vi "RTG Example_reduced_20230830.vi"() -> ()   [LabVIEW 2020]
doc: "This example illustrates how to use the RTG local API to control the RTG."
uses:
  <vilib>/RTG/API/ip/common/host-types/Target Configuration.ctl
  <vilib>/RTG/API/ip/common/host-types/Synchronization - Host.ctl
  <vilib>/RTG/API/ip/common/host-types/Synchronization Mode - Host.ctl
  <vilib>/RTG/API/ip/common/host-types/Basic Target - Host.ctl
  <vilib>/RTG/API/interface/public/State.ctl
  <vilib>/RTG/coprocessor/host/RTG Coprocessor Link Interface/Public/Coprocessor Status.ctl
  <vilib>/RTG/API/ip/common/host-types/Target Motion Parameters.ctl
  <vilib>/RTG/API/ip/common/host-types/Single Target Motion Parameters.ctl
  <vilib>/RTG/API/interface/public/Coprocessor Link Status.ctl
  support/Options - API Mode.ctl
  support/Options - Calibration.ctl
  support/Options - Remote.ctl
  <vilib>/Utility/error.llb/Error Cluster From Error Code.vi
  <vilib>/rvi/errors/niLvFpgaAdjustHostInterfaceError.vi
  <vilib>/rvi/interface/nirviReadWriteControl/nirviReadWriteControl.xnode
  <vilib>/RTG/API/interface/NI-RTG Interface.lvclass
  <vilib>/RTG/coprocessor/host/RTG Coprocessor Link Interface/RTG Coprocessor Link Interface.lvclass
  <vilib>/RTG/API/ip/common/host-types/Host Data Types v1.lvlib
  RTG Examples.lvlib
  NiFpgaLv.dll
  <vilib>/rvi/interface/Simulation/niFpgaSimulationCallBeginRW.vi
panel:
  out "RTG Status":string
  out "RTG State":T1
  in  "tab":T2(tab)
  in  "abort system self cal":bool
  in  "Set PRIs":bool
  in  "PRI (s)":dbl[](array[numeric]) format="%#_6p"
  in  "Calibrate":bool=TRUE
  in  "Instrument Names":string[](array[string])=["5831_0"]
  in  "Center Freqeuncies (Hz)":dbl[](array[numeric])=[5500000000.0] format="%#_6p"
  in  "Reference Levels (dBm)":dbl[](array[numeric])=[0.0]
  in  "mmWave Radio Heads Enable":bool[](array[boolean])
  in  "External Delay (s)":dbl[](array[numeric]) format="%#_6p"
  in  "External Attenuations (dB)":dbl[](array[numeric])
  in  "Offset Frequencies (Hz)":dbl[](array[numeric]) format="%#_6p"
  out "Error Out":errorcluster caption="error out"
  in  "Coprocessor Names":string[](array[string])
  out "Versions":string[](array[string])
  out "Max Common Attenuations (dB)":dbl[](array[numeric])
  out "Min Common Attenuations (dB)":dbl[](array[numeric])
  out "Min Latencies (s)":dbl[](array[numeric]) format="%#_6p"
  in  "configure common attenuation":bool
  in  "Common Attenuation (dB)":dbl
  in  "set hardware trigger":bool
  in  "send target motion":bool
  in  "Auto Send Software Trigger":bool
  in  "Prepend Software Trigger":bool
  in  "send files":bool
  in  "Target Configuration Files":path[](array[path])
  in  "pulse detection calibration":bool
  in  "send target config":bool
  in  "send sw trigger":bool
  in  "start rtg":bool
  in  "stop rtg":bool
  in  "abort":bool
  in  "Target Configuration":T3 {"rtg targets"."time offset (s)" format="%#_6p"; "rtg targets"."doppler" format="%#_6p"}
  in  "Device Index":i32
  in  "Target Motion Parameters":T7={"target motions"=[{"target enable"=FALSE, "start time offset (s)"=-1e-09, "time offset rate of change (s/s)"=0.001, "start attenuation (dB)"=0.0, "attenuation rate of change (dB/s)"=0.0, "start frequency shift (Hz)"=0.0, "frequency shift rate of change (Hz/sec)"=0.0}], "scenario duration (s)"=67.0, "configuration update rate(Hz)"=15000.0} {"configuration update rate(Hz)" format="%#_6p"; "target motions"."frequency shift rate of change (Hz/sec)" format="%#_6p"; "target motions"."start frequency shift (Hz)" format="%#_6p"; "target motions"."time offset rate of change (s/s)" format="%#_6p"; "target motions"."start time offset (s)" format="%#_6p"}
  in  "Data Path Enable":bool=TRUE
  in  "Hardware Trigger":string="PXI_Trig7"
  out "Device Index vs Trigger Count":i32[][](array[numeric])
  out "coprocessor link status":T9[](array[typedef])
  out "rtg link status":T10[](array[typedef])
  # "Coprocessor"
  # "Configuration Files and Target Motion"
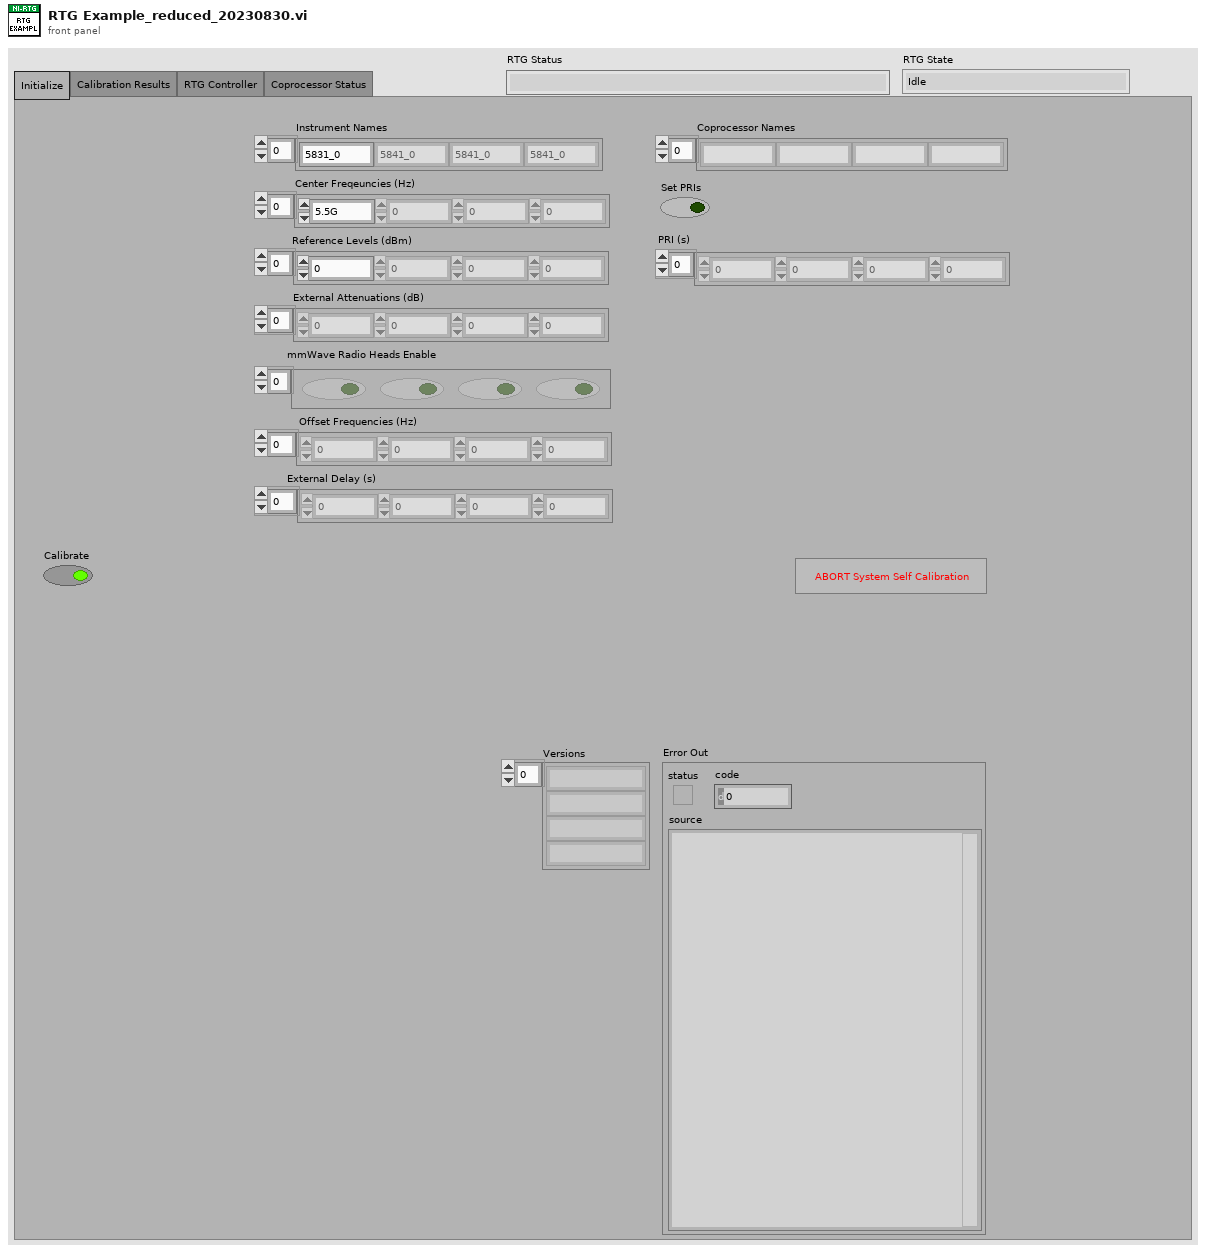
[diagram p1: front panel]
types:
  T1 = typedef "NI-RTG v1.lvlib/NI-RTG Interface.lvclass/State.ctl" = enum16{"Idle", "Inactive", "Active", "System Self Calibration"}
  T2 = enum32{"Initialize", "Calibration Results", "RTG Controller", "Coprocessor Status"}
  T3 = typedef "Host Data Types v1.lvlib/Target Configuration.ctl" = cluster{"synchronization":T4, "rtg targets":T6[]}
  T4 = typedef "Host Data Types v1.lvlib/Synchronization - Host.ctl" = cluster{"synch mode":T5, "time offset (s)":dbl}
  T5 = typedef "Host Data Types v1.lvlib/Synchronization Mode - Host.ctl" = enum16{"Software Trigger", "Hardware Trigger", "Time Offset Relative to First", "Time Offset Relative to Last", "Pulse Rising Edge", "Pulse Falling Edge"}
  T6 = typedef "Host Data Types v1.lvlib/Basic Target - Host.ctl" = cluster{"time offset (s)":dbl, "attenuaton (dB)":dbl, "doppler":dbl, "target enable":bool, "relative velocity enable":bool}
  T7 = typedef "Host Data Types v1.lvlib/Target Motion Parameters.ctl" = cluster{"target motions":T8[], "scenario duration (s)":dbl, "configuration update rate(Hz)":dbl}
  T8 = typedef "Host Data Types v1.lvlib/Single Target Motion Parameters.ctl" = cluster{"target enable":bool, "start time offset (s)":dbl, "time offset rate of change (s/s)":dbl, "start attenuation (dB)":dbl, "attenuation rate of change (dB/s)":dbl, "start frequency shift (Hz)":dbl, "frequency shift rate of change (Hz/sec)":dbl}
  T9 = typedef "RTG Coprocessor Link Interface v1 Host.lvlib/RTG Coprocessor Link Interface.lvclass/Coprocessor Status.ctl" = cluster{"tx read count":u64, "tx read overflow":bool, "rx read count":u64, "rx read overflow":bool}
  T10 = typedef "NI-RTG v1.lvlib/NI-RTG Interface.lvclass/Coprocessor Link Status.ctl" = cluster{"task name":string, "device name":string, "hard error":bool, "soft error":bool, "channel up":bool, "system reset":bool}
  T11 = typedef "RTG Examples.lvlib/Options - API Mode.ctl" = enum16{"Local", "Remote"}
  T12 = typedef "RTG Examples.lvlib/Options - Calibration.ctl" = cluster{"enable internal loopback  ":bool, "enable overwrite cal data  ":bool, "enable save cal data           ":bool, "disable self cal range          ":bool}
  T13 = typedef "RTG Examples.lvlib/Options - Remote.ctl" = cluster{"ip address":string, "port":string, "certificate path":path, "timeout (ms)":i32}
  T14 = cluster{"API Mode":T11, "Calibration Options":T12, "Remote Options":T13, "ini file path":path}
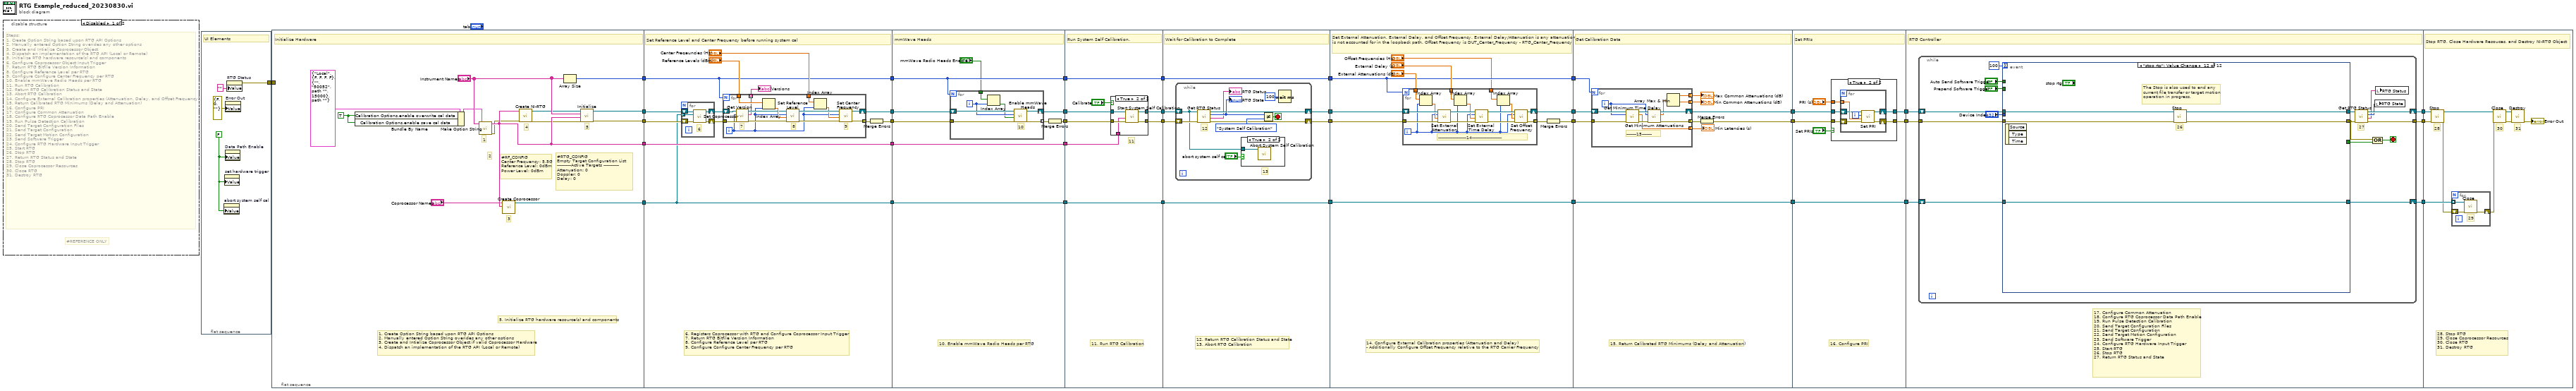
[diagram p0: block diagram]
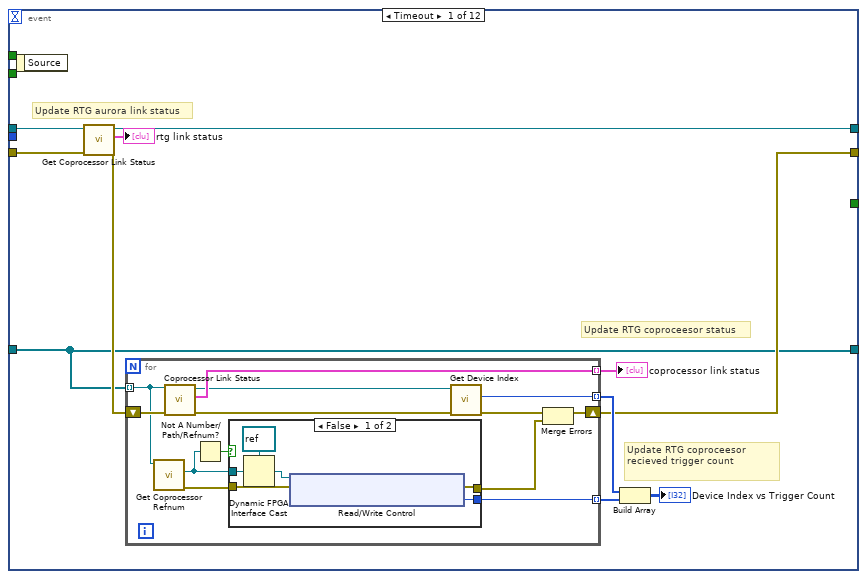
[diagram p6: hidden frame]
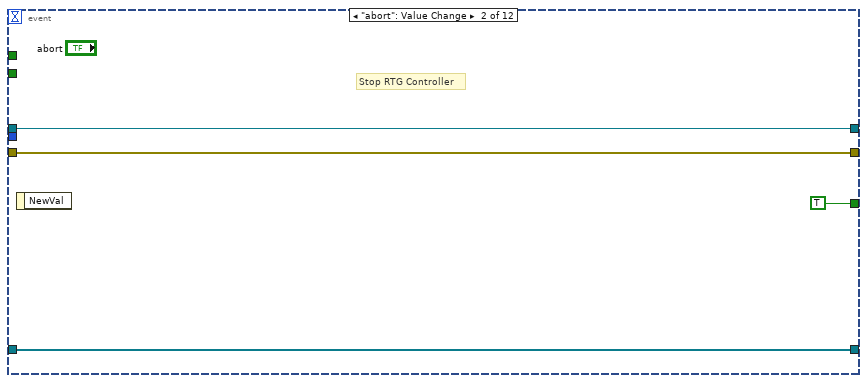
[diagram p8: hidden frame]
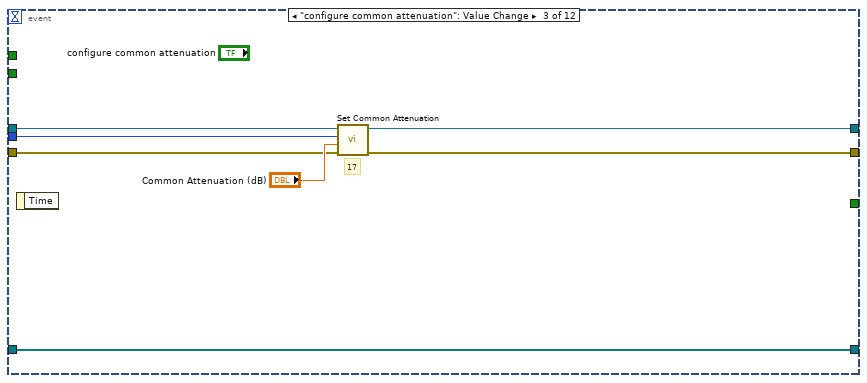
[diagram p9: hidden frame]
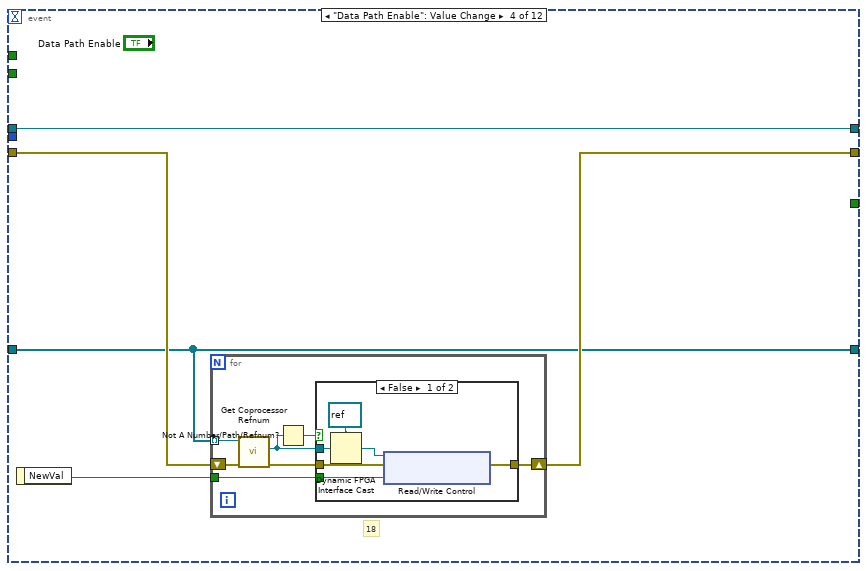
[diagram p10: hidden frame]
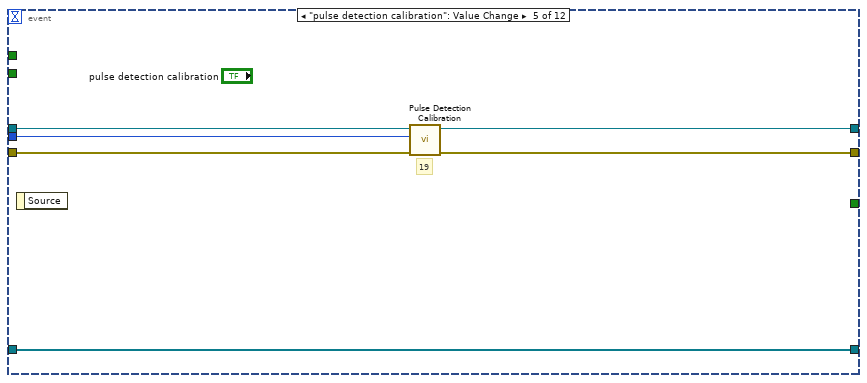
[diagram p12: hidden frame]
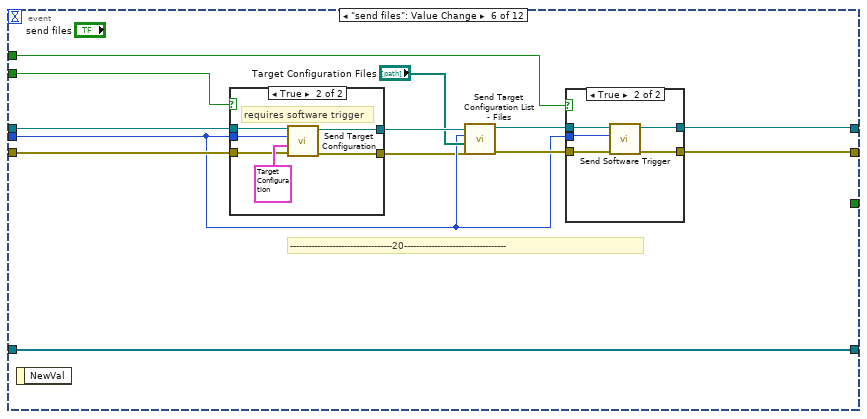
[diagram p13: hidden frame]
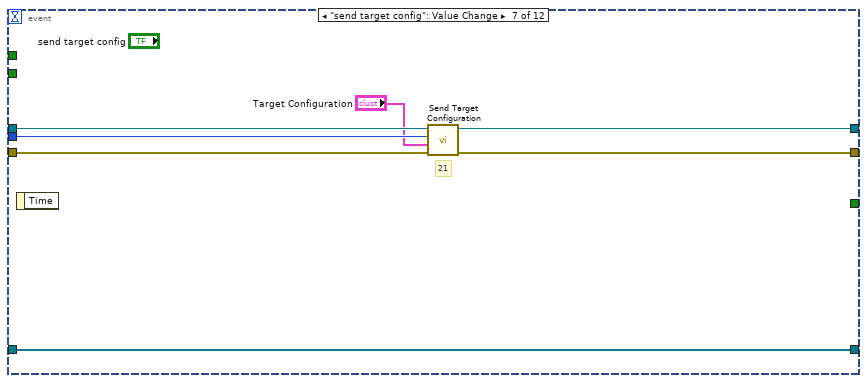
[diagram p16: hidden frame]
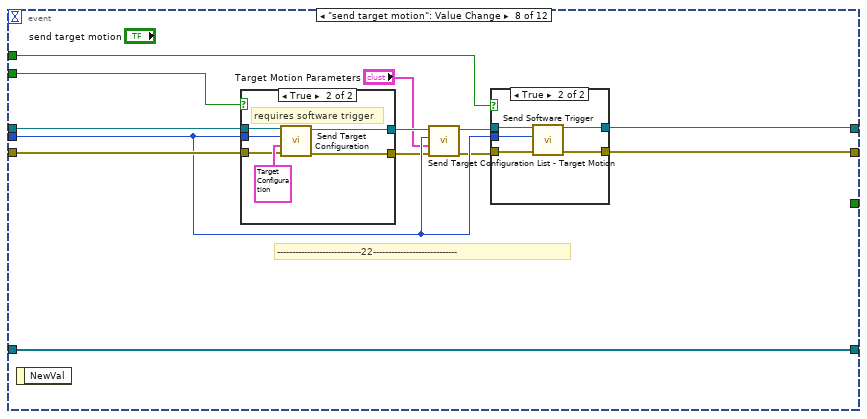
[diagram p17: hidden frame]
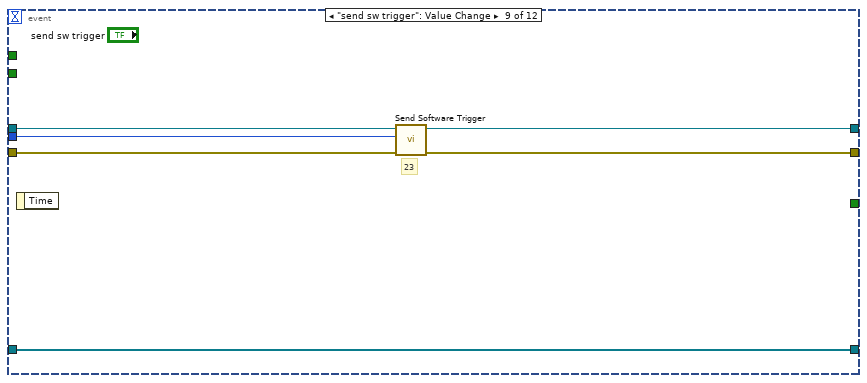
[diagram p20: hidden frame]
diagram:
  n1 = disable-structure shown="Disabled" {
    frame Disabled {
      # "#REFERENCE ONLY"
      # "Steps:\n1. Create Option String based upon RTG API Options\n2. Manually entered Option String overides any other options\n3. Create and Intialize Coprocessor Object\n4. Dispatch an implementation of the RTG API (Local or Remote)\n5. Initialize RTG hardware resource(s) and components\n6. Configure Coprocessor Object Input Trigger\n7. Return RTG Bitfile Version Information\n8. Configure Reference Level per RTG\n9. Configure Configure Center Frequency per RTG\n10. Enable mmWave Radio Heads per RTG\n11. Run RTG Calibration\n12. Return RTG Calibration Status and State\n13. Abort RTG Calibration\n14. Configure External Calibration properties (Attenuation, Delay, and Offset Frequency)\n15. Return Calibrated RTG Minimums (Delay and Attenuation)\n16. Configure PRI\n17. Configure Common Attenuation\n18. Configure RTG Coprocessor Data Path Enable \n19. Run Pulse Detection Calibration\n20. Send Target Configuration Files\n21. Send Target Configuration\n22. Send Target Motion Configuration\n23. Send Software Trigger\n24. Configure RTG Hardware Input Trigger\n25. Start RTG\n26. Stop RTG\n27. Return RTG Status and State\n28. Stop RTG\n29. Close Coprocessor Resources\n30. Close RTG\n31. Destroy RTG"
    }
    frame Enabled {
    }
  }
  n2 = flat-sequence {
    tunnel: [w40] -> w7
    frame #0 {
      w38 = FALSE ("bitfiles loaded")
      # "UI Elements"
      n3 = property on="abort system self cal" class="Bool (strict)"("Value"=w38) -> ()  [unwired: 2 in, 2 out]
      n4 = property on="set hardware trigger" class="Bool (strict)"("Value"=w38) -> ()  [unwired: 2 in, 2 out]
      n5 = property on="Data Path Enable" class="Bool (strict)"("Value"=w38) -> ()  [unwired: 2 in, 2 out]
      n6 = property on="Error Out" class="Clust (strict)"("Value"=errorcluster {"status"=FALSE, "code"=0, "source"=""} ("error out")) -> ()  [unwired: 2 in, 2 out]
      n7 = property on="RTG Status" class="Str"("Value"="" ("rtg status")) -> (error out=w40:errorcluster)  [unwired: 2 in, 1 out]
    }
  }
  n8 = flat-sequence {
    tunnel: [w49] -> w37
    tunnel: [w47] -> w36
    tunnel: [w54] -> w35
    tunnel: [w52] -> w17
    tunnel: [w51] -> w14
    tunnel: w7 -> [_]
    tunnel: w37 -> [w58]
    tunnel: w36 -> [w55]
    tunnel: [w65] -> w29
    tunnel: [w63] -> w27
    tunnel: w35 -> [w62]
    tunnel: [w62] -> w25
    tunnel: w17 -> [w61]
    tunnel: [w61] -> w16
    tunnel: w14 -> [w57]
    tunnel: [w57] -> w12
    tunnel: w29 -> [w94]
    tunnel: [w89] -> w28
    tunnel: w27 -> [w93]
    tunnel: [w91] -> w26
    tunnel: w25 -> [w95]
    tunnel: [w95] -> w24
    tunnel: w16 -> [w88]
    tunnel: [w88] -> w15
    tunnel: [w87] -> w13
    tunnel: w12 -> [w87]
    tunnel: w28 -> [w110]
    tunnel: w26 -> [w109]
    tunnel: [w107] -> w23
    tunnel: [w108] -> w22
    tunnel: w24 -> [w108]
    tunnel: [w106] -> w20
    tunnel: w15 -> [w105]
    tunnel: w13 -> [w103]
    tunnel: [w103] -> w11
    tunnel: w23 -> [w122]
    tunnel: w22 -> [w123]
    tunnel: [w123] -> w21
    tunnel: w20 -> [w121]
    tunnel: [w120] -> w19
    tunnel: [w119] -> w18
    tunnel: w11 -> [w118]
    tunnel: [w118] -> w10
    tunnel: [w141] -> w32
    tunnel: [w140] -> w31
    tunnel: [w139] -> w30
    tunnel: w21 -> [w139]
    tunnel: w19 -> [w138]
    tunnel: w18 -> [w137]
    tunnel: w10 -> [w135]
    tunnel: [w135] -> w9
    tunnel: w32 -> [w167]
    tunnel: [w166] -> w6
    tunnel: w31 -> [w169]
    tunnel: [w165] -> w4
    tunnel: w30 -> [w161]
    tunnel: w9 -> [w160]
    tunnel: [w160] -> w2
    tunnel: w6 -> [w185]
    tunnel: [w184] -> w5
    tunnel: w4 -> [w183]
    tunnel: [w182] -> w3
    tunnel: w2 -> [w187]
    tunnel: [w187] -> w1
    tunnel: w5 -> [w206]
    tunnel: w3 -> [w205]
    tunnel: [w204] -> w34
    tunnel: [w203] -> w33
    tunnel: w1 -> [w202]
    tunnel: [w201] -> w8
    tunnel: w34 -> [w395]
    tunnel: w33 -> [w389]
    tunnel: w8 -> [w390]
    frame #0 {
      w42 = TRUE ("Calibration Options.enable overwrite cal data")
      # "1. Create Option String based upon RTG API Options\n2. Manually entered Option String overides any other options\n3. Create and Intialize Coprocessor Object if valid Coprocessor Hardware\n4. Dispatch an implementation of the RTG API (Local or Remote)"
      # "4"
      # "3"
      # "2"
      # "1"
      # "5. Initialize RTG hardware resource(s) and components"
      # "5"
      # "#RTG_CONFIG\nEmpty Target Configuration List\n----------Active Targets -----------\nAttenuation: 0\nDoppler: 0\nDelay: 0"
      # "#RF_CONFIG\nCenter Frequency: 5.5G\nReference Level: 0dBm\nPower Level: 0dBm"
      # "Initialize Hardware"
      n9 = Bundle By Name(cluster=T14 {"API Mode"=enum."Local", "Calibration Options"={"enable internal loopback  "=FALSE, "enable overwrite cal data  "=FALSE, "enable save cal data           "=FALSE, "disable self cal range          "=FALSE}, "Remote Options"={"ip address"="", "port"="50052", "certificate path"=path "", "timeout (ms)"=15000}, "ini file path"=path ""} ("RTG API Options"), "Calibration Options.enable overwrite cal data"=w42, "Calibration Options.enable save cal data"=w42) -> (w43:T14)
      n10 = call "Make Option String.vi"("RTG API Options"=w43, "instrument names"="Instrument Names") -> ("error out"=w45:errorcluster, "option string"=w52:string)  [unwired: 8 in]
      n11 = call <vilib>:"Create Coprocessor.vi"("option string"=w52, "coprocessor resources"="Coprocessor Names") -> ("rtg coprocessor links"=w51:refnum<class "RTG Coprocessor Link Interface.lvclass">[])  [unwired: 8 in, 1 out]
      n12 = call <vilib>:"Create NI-RTG.vi"("error in"=w45, "option string"=w52) -> ("error out"=w48:errorcluster, "NI-RTG Interface out"=w50:refnum<class "NI-RTG Interface.lvclass">)  [unwired: 8 in]
      n13 = Array Size(array="Instrument Names") -> (size(s)=w54:i32)
      n14 = call-dynamic "Initialize.vi"("error in"=w48, "option string"=w52, "instrument names"="Instrument Names", "ni-rtg interface"=w50) -> ("error out"=w49:errorcluster, "ni-rtg interface out"=w47:refnum<class "NI-RTG Interface.lvclass">)  [unwired: 6 in]
    }
    frame #1 {
      # "6. Registers Coprocessor with RTG and Configure Coprocessor Input Trigger\n7. Return RTG Bitfile Version Information\n8. Configure Reference Level per RTG\n9. Configure Configure Center Frequency per RTG"
      # "Set Reference Level and Center Frequency before running system cal"
      n15 = for {
        shift-right: [w86] -> w60
        shift-left: w58 -> [w84]
        shift-right: [w85] -> w59
        shift-left: w55 -> [w83]
        tunnel: w57 -> [w82] mode=indexing
        # "6"
        n16 = call-dynamic "Set Coprocessor.vi"("error in"=w84, "rtg coprocessor link interface"=w82, "rtg api interface"=w83) -> ("error out"=w86:errorcluster, "rtg api interface out"=w85:refnum<class "NI-RTG Interface.lvclass">)  [unwired: 7 in]
      }
      n17 = for {
        N: w62 -> [_]
        tunnel: w60 -> [w71]
        tunnel: "Reference Levels (dBm)" -> [w79]
        tunnel: "Center Freqeuncies (Hz)" -> [w77]
        shift-right: [w75] -> w65
        shift-left: w59 -> [w73]
        tunnel: [w74] -> w64 mode=indexing
        tunnel: [w68] -> w56 mode=indexing
        i -> [w69]
        # "9"
        # "8"
        # "7"
        n18 = call-dynamic "Get Version.vi"("error in"=w71, "device index (0)"=w69, "NI-RTG Interface in"=w73) -> ("error out"=w70:errorcluster, "version"=w68:string, "NI-RTG Interface out"=w72:refnum<class "NI-RTG Interface.lvclass">)  [unwired: 6 in]
        n19 = Index Array(array=w79, index=w69) -> (element=w78:dbl)
        n20 = call-dynamic "Set Reference Level.vi"("error in"=w70, "reference level (dBm)"=w78, "device index (0)"=w69, "rtg api interface"=w72) -> ("error out"=w80:errorcluster, "rtg api interface out"=w81:refnum<class "NI-RTG Interface.lvclass">)  [unwired: 6 in]
        n21 = Index Array(array=w77, index=w69) -> (element=w76:dbl)
        n22 = call-dynamic "Set Center Frequency.vi"("error in"=w80, "center frequency (Hz)"=w76, "device index (0)"=w69, "rtg api interface"=w81) -> ("error out"=w74:errorcluster, "rtg api interface out"=w75:refnum<class "NI-RTG Interface.lvclass">)  [unwired: 6 in]
      }
      "Versions" <- w56
      n23 = Merge Errors(w64) -> (w63:errorcluster)
    }
    frame #2 {
      # "10. Enable mmWave Radio Heads per RTG"
      # "mmWave Heads"
      n24 = for {
        N: w95 -> [_]
        shift-right: [w99] -> w89
        shift-left: w94 -> [w100]
        tunnel: w93 -> [w102]
        tunnel: [w101] -> w92 mode=indexing
        tunnel: "mmWave Radio Heads Enable" -> [w98]
        i -> [w97]
        # "10"
        n25 = Index Array(array=w98, index=w97) -> (element=w96:bool)
        n26 = call-dynamic "Enable mmWave Heads.vi"("error in"=w102, "enable mmWave"=w96, "device index (0)"=w97, "ni-rtg interface"=w100) -> ("error out"=w101:errorcluster, "ni-rtg interface out"=w99:refnum<class "NI-RTG Interface.lvclass">)  [unwired: 6 in]
      }
      n27 = Merge Errors(w92) -> (w91:errorcluster)
    }
    frame #3 {
      # "11. Run RTG Calibration"
      # "11"
      # "Run System Self Calibration."
      n28 = case shown="True" "Calibrate" {
        tunnel: w110 -> [w112 w117]
        tunnel: w109 -> [w111 w116]
        tunnel: [w112 w115] -> w107
        tunnel: [w111 w114] -> w106
        tunnel: w105 -> [_ w113]
        frame False {
        }
        frame True {
          n29 = call-dynamic "Start System Self Calibration.vi"("error in"=w116, "option string"=w113, "rtg api interface"=w117) -> ("error out"=w114:errorcluster, "rtg api interface out"=w115:refnum<class "NI-RTG Interface.lvclass">)  [unwired: 7 in]
        }
      }
    }
    frame #4 {
      # "12. Return RTG Calibration Status and State\n13. Abort RTG Calibration"
      # "Wait for Calibration to Complete"
      n30 = while {
        shift-right: [w129] -> w120
        shift-left: w122 -> [w125]
        shift-right: [w130] -> w119
        shift-left: w121 -> [w133]
        stop <- w128 stop-if-true
        # "13"
        # "12"
        n31 = call-dynamic "Get RTG Status.vi"("error in"=w133, "rtg api interface"=w125) -> ("error out"=w130:errorcluster, "rtg status"=→"RTG Status":string, "state"=w132:T1, "rtg api interface out"=w129:refnum<class "NI-RTG Interface.lvclass">)  [unwired: 6 in]
        "RTG State" <- w132
        n32 = case shown="True" "abort system self cal" {
          tunnel: w125 -> [_ w134]
          frame False {
          }
          frame True {
            n33 = call-dynamic "Abort System Self Calibration.vi"("rtg-api interface"=w134) -> ()  [unwired: 9 in, 2 out]
          }
        }
        n34 = Not Equal?(x=w132, y=State."System Self Calibration") -> (x != y?=w128:bool)
        n35 = Wait (ms)(milliseconds to wait=u32 100) -> ()  [unwired: 1 out]
      }
    }
    frame #5 {
      # "14. Configure External Calibration properties (Attenuation and Delay)\n- Additionally Configure Offset Frequency relative to the RTG Carrier Frequency"
      # "Set External Attenuation, External Delay, and Offset Frequency. External Delay/Attenuation is any attenuation/delay that is not accounted for in the loopback path. Offset Frequency is DUT_Center_Frequency - RTG_Center_Frequency"
      n36 = for {
        N: w139 -> [_]
        shift-right: [w149] -> w141
        shift-left: w138 -> [w159]
        tunnel: "External Attenuations (dB)" -> [w157]
        tunnel: "External Delay (s)" -> [w155]
        tunnel: [w151] -> w142 mode=indexing
        tunnel: w137 -> [w148]
        tunnel: "Offset Frequencies (Hz)" -> [w147]
        i -> [w145]
        # "--------------------14---------------------"
        n37 = Index Array(array=w157, index=w145) -> (element=w156:dbl)
        n38 = call-dynamic "Set External Attenuation.vi"("error in"=w148, "external attenuation (dB)"=w156, "device index (0)"=w145, "rtg api interface"=w159) -> ("error out"=w153:errorcluster, "rtg api interface out"=w158:refnum<class "NI-RTG Interface.lvclass">)  [unwired: 6 in]
        n39 = Index Array(array=w155, index=w145) -> (element=w154:dbl)
        n40 = call-dynamic "Set External Time Delay.vi"("error in"=w153, "delay (s)"=w154, "device index (0)"=w145, "rtg api interface"=w158) -> ("error out"=w152:errorcluster, "rtg api interface out"=w150:refnum<class "NI-RTG Interface.lvclass">)  [unwired: 6 in]
        n41 = Index Array(array=w147, index=w145) -> (element=w146:dbl)
        n42 = call-dynamic "Set Offset Frequency.vi"("error in"=w152, "offset frequency (Hz)"=w146, "device index (0)"=w145, "NI-RTG Interface in"=w150) -> ("error out"=w151:errorcluster, "NI-RTG Interface out"=w149:refnum<class "NI-RTG Interface.lvclass">)  [unwired: 6 in]
      }
      n43 = Merge Errors(w142) -> (w140:errorcluster)
    }
    frame #6 {
      # "15. Return Calibrated RTG Minimums (Delay and Attenuation)"
      # "Get Calibration Data"
      n44 = for {
        N: w161 -> [_]
        tunnel: w169 -> [w180]
        tunnel: [w177] -> w168 mode=indexing
        shift-right: [w175] -> w166
        shift-left: w167 -> [w178]
        tunnel: [w174] -> w162 mode=indexing
        tunnel: [w172] -> w164 mode=indexing
        tunnel: [w171] -> w163 mode=indexing
        i -> [w170]
        # "-------15-------"
        n45 = call-dynamic "Get Minimum Time Delay.vi"("error in"=w180, "device index (0)"=w170, "rtg api interface"=w178) -> ("error out"=w179:errorcluster, "delay (s)"=w174:dbl, "rtg api interface out"=w176:refnum<class "NI-RTG Interface.lvclass">)  [unwired: 5 in, 1 out]
        n46 = call-dynamic "Get Minimum Attenuations.vi"("error in"=w179, "device index (0)"=w170, "rtg api interface"=w176) -> ("error out"=w177:errorcluster, "attenuations (dB)"=w173:dbl[], "rtg api interface out"=w175:refnum<class "NI-RTG Interface.lvclass">)  [unwired: 5 in, 1 out]
        n47 = Array Max & Min(array=w173) -> (max value=w172:dbl, min value=w171:dbl)  [unwired: 2 out]
      }
      "Max Common Attenuations (dB)" <- w164
      "Min Common Attenuations (dB)" <- w163
      "Min Latencies (s)" <- w162
      n48 = Merge Errors(w168) -> (w165:errorcluster)
    }
    frame #7 {
      # "16. Configure PRI"
      # "Set PRIs"
      n49 = case shown="True" "Set PRIs" {
        tunnel: w185 -> [w189 w191]
        tunnel: [w189 w193] -> w184
        tunnel: w183 -> [w188 w190]
        tunnel: [w188 w192] -> w182
        tunnel: "PRI (s)" -> [_ w194]
        frame False {
        }
        frame True {
          n50 = for {
            tunnel: w194 -> [w200] mode=indexing
            shift-right: [w198] -> w193
            shift-left: w191 -> [w196]
            shift-right: [w197] -> w192
            shift-left: w190 -> [w195]
            i -> [w199]
            n51 = call-dynamic "Set PRI.vi"("error in"=w195, "pri (s)"=w200, "device index (0)"=w199, "NI-RTG Interface in"=w196) -> ("error out"=w197:errorcluster, "NI-RTG Interface out"=w198:refnum<class "NI-RTG Interface.lvclass">)  [unwired: 6 in]
          }
        }
      }
    }
    frame #8 {
      # "17. Configure Common Attenuation\n18. Configure RTG Coprocessor Data Path Enable \n19. Run Pulse Detection Calibration\n20. Send Target Configuration Files\n21. Send Target Configuration\n22. Send Target Motion Configuration\n23. Send Software Trigger\n24. Configure RTG Hardware Input Trigger\n25. Start RTG\n26. Stop RTG\n27. Return RTG Status and State"
      # "RTG Controller"
      n52 = while {
        tunnel: w205 -> [w221]
        shift-right: [w217] -> w204
        shift-left: w206 -> [w222]
        tunnel: [w216] -> w203
        shift-right: [w212] -> w201
        shift-left: w202 -> [w213]
        stop <- w210 stop-if-true
        # "27"
        n53 = event shown="[11] \"stop rtg\": Value Change" {
          selector: _ -> [_ _ _ _ _ _ _ _ _ _ _ _]
          dyn-events: _ -> [_ _ _ _ _ _ _ _ _ _ _ _]
          timeout: 100 -> [_ _ _ _ _ _ _ _ _ _ _ _]
          tunnel: [_ TRUE _ _ _ _ _ _ _ _ _ _] -> w220
          tunnel: w222 -> [w233 w256 w264 w269 w287 w301 w324 w336 w358 w364 w381 w386]
          tunnel: w221 -> [w225 w255 w259 w267 w285 w300 w319 w335 w354 w363 w378 w383]
          tunnel: [w232 w256 w263 w269 w288 w296 w323 w334 w357 w365 w380 w385] -> w218
          tunnel: [w224 w255 w258 w266 w284 w292 w318 w327 w353 w359 w377 w382] -> w209
          tunnel: "Device Index" -> [_ _ w262 _ w289 w294 w322 w333 w356 w362 _ _]
          tunnel: w213 -> [w223 w254 w260 w265 w286 w302 w320 w337 w355 w360 w379 w384]
          tunnel: [w223 w254 w260 w265 w286 w302 w320 w337 w355 w360 w379 w384] -> w212
          tunnel: "Auto Send Software Trigger" -> [_ _ _ _ _ w291 _ w325 _ _ _ _]
          tunnel: "Prepend Software Trigger" -> [_ _ _ _ _ w290 _ w326 _ _ _ _]
          event Timeout {
            # "Update RTG coproceesor \nrecieved trigger count"
            # "Update RTG coproceesor status"
            # "Update RTG aurora link status"
            n54 = event-data() -> ()  [unwired: 1 in, 1 out]
            n55 = call-dynamic "Get Coprocessor Link Status.vi"("error in"=w225, "rtg api interface"=w233) -> ("error out"=w231:errorcluster, "rtg link status"=→"rtg link status":T10[], "rtg api interface out"=w232:refnum<class "NI-RTG Interface.lvclass">)  [unwired: 7 in]
            n56 = for {
              tunnel: w223 -> [w241] mode=indexing
              tunnel: [w245] -> w230 mode=indexing
              shift-right: [w238] -> w224
              shift-left: w231 -> [w246]
              tunnel: [w240] -> w228 mode=indexing
              tunnel: [w234] -> w229 mode=indexing
              n57 = call-dynamic "Get Coprocessor Refnum.vi"("rtg coprocessor link interface"=w241) -> ("error out"=w244:errorcluster, "coprocessor refnum"=w242:refnum<k20>)  [unwired: 8 in, 1 out]
              n58 = call-dynamic "Coprocessor Link Status.vi"("error in"=w246, "rtg coprocessor link interface"=w241) -> ("error out"=w236:errorcluster, "coprocessor status out"=w245:T9, "rtg coprocessor link interface out"=w237:refnum<class "RTG Coprocessor Link Interface.lvclass">)  [unwired: 7 in]
              n59 = Not A Number/Path/Refnum?(number/path/refnum=w242) -> (NaN/Path/Refnum?=w243:bool)
              n60 = case shown="False" w243 {
                tunnel: w242 -> [w250 _]
                tunnel: w244 -> [w249 w253]
                tunnel: [w248 w253] -> w239
                tunnel: [w247 _] -> w240
                frame False {
                  n61 = Dynamic FPGA Interface Cast(Session In=refnum<k20> refnum ("Type"), Type=w250) -> (Session Out=w252:refnum<k20>)
                  n62 = xnode "Read/Write Control"("FPGA VI Reference In"=w252, "error in"=w249) -> ("error out"=w248:errorcluster, "read trigger rising edge count"=w247:u16)  [unwired: 1 out]
                }
                frame True {
                }
              }
              n63 = call-dynamic "Get Device Index.vi"("error in"=w236, "rtg coprocessor link interface"=w237) -> ("error out"=w235:errorcluster, "device index"=w234:i32)  [unwired: 7 in, 1 out]
              n64 = Merge Errors(w235, w239) -> (w238:errorcluster)
            }
            "coprocessor link status" <- w230
            n65 = Build Array(w229, w228) -> (→"Device Index vs Trigger Count":i32[][])
          }
          event "abort": Value Change {
            # "Stop RTG Controller"
            n66 = event-data() -> ()  [unwired: 1 in, 1 out]
          }
          event "configure common attenuation": Value Change {
            # "17"
            n67 = event-data() -> ()  [unwired: 1 in, 1 out]
            n68 = call-dynamic "Set Common Attenuation.vi"("error in"=w259, "attenuation (dB)"="Common Attenuation (dB)", "device index (0)"=w262, "rtg api interface"=w264) -> ("error out"=w258:errorcluster, "rtg api interface out"=w263:refnum<class "NI-RTG Interface.lvclass">)  [unwired: 5 in, 1 out]
          }
          event "Data Path Enable": Value Change {
            # "18"
            n69 = event-data() -> ("NewVal"=w268:bool)  [unwired: 1 in]
            n70 = for {
              tunnel: w265 -> [w276] mode=indexing
              tunnel: w268 -> [w273]
              shift-right: [w271] -> w266
              shift-left: w267 -> [w270]
              n71 = call-dynamic "Get Coprocessor Refnum.vi"("error in"=w270, "rtg coprocessor link interface"=w276) -> ("error out"=w272:errorcluster, "coprocessor refnum"=w275:refnum<k20>)  [unwired: 7 in, 1 out]
              n72 = Not A Number/Path/Refnum?(number/path/refnum=w275) -> (NaN/Path/Refnum?=w274:bool)
              n73 = case shown="False" w274 {
                tunnel: w275 -> [w280 _]
                tunnel: w273 -> [w279 _]
                tunnel: w272 -> [w278 w283]
                tunnel: [w277 w283] -> w271
                frame False {
                  n74 = Dynamic FPGA Interface Cast(Session In=refnum<k20> refnum ("Type"), Type=w280) -> (Session Out=w282:refnum<k20>)
                  n75 = xnode "Read/Write Control"("FPGA VI Reference In"=w282, "error in"=w278, "data path enable"=w279) -> ("error out"=w277:errorcluster)  [unwired: 1 out]
                }
                frame True {
                }
              }
            }
          }
          event "pulse detection calibration": Value Change {
            # "19"
            n76 = event-data() -> ()  [unwired: 1 in, 1 out]
            n77 = call-dynamic "Pulse Detection Calibration.vi"("error in"=w285, "device index (0)"=w289, "rtg api interface"=w287) -> ("error out"=w284:errorcluster, "rtg api interface out"=w288:refnum<class "NI-RTG Interface.lvclass">)  [unwired: 7 in]
          }
          event "send files": Value Change {
            # "----------------------------------20----------------------------------"
            n78 = event-data() -> ()  [unwired: 1 in, 1 out]
            n79 = case shown="True" w290 {
              tunnel: w301 -> [w311 w316]
              tunnel: w300 -> [w310 w313]
              tunnel: w294 -> [_ w315]
              tunnel: [w311 w314] -> w299
              tunnel: [w310 w312] -> w293
              frame False {
              }
              frame True {
                # "requires software trigger"
                n80 = call-dynamic "Send Target Configuration.vi"("error in"=w313, "target config"=T3 {"synchronization"={"synch mode"=enum."Software Trigger", "time offset (s)"=0.0}, "rtg targets"=[{"time offset (s)"=0.0, "attenuaton (dB)"=0.0, "doppler"=0.0, "target enable"=FALSE, "relative velocity enable"=FALSE}, {"time offset (s)"=0.0, "attenuaton (dB)"=0.0, "doppler"=0.0, "target enable"=FALSE, "relative velocity enable"=FALSE}, {"time offset (s)"=0.0, "attenuaton (dB)"=0.0, "doppler"=0.0, "target enable"=FALSE, "relative velocity enable"=FALSE}, {"time offset (s)"=0.0, "attenuaton (dB)"=0.0, "doppler"=0.0, "target enable"=FALSE, "relative velocity enable"=FALSE}]}, "device index (0)"=w315, "rtg api interface"=w316) -> ("error out"=w312:errorcluster, "rtg api interface out"=w314:refnum<class "NI-RTG Interface.lvclass">)  [unwired: 5 in, 1 out]
              }
            }
            n81 = call-dynamic "Send Target Configuration List - Files.vi"("error in"=w293, "target configuration file path"="Target Configuration Files", "device index (0)"=w294, "rtg api interface"=w299) -> ("error out"=w295:errorcluster, "rtg api interface out"=w297:refnum<class "NI-RTG Interface.lvclass">)  [unwired: 6 in]
            n82 = case shown="True" w291 {
              tunnel: w297 -> [w304 w309]
              tunnel: [w304 w308] -> w296
              tunnel: w295 -> [w303 w307]
              tunnel: [w303 w306] -> w292
              tunnel: w294 -> [_ w305]
              frame False {
              }
              frame True {
                n83 = call-dynamic "Send Software Trigger.vi"("error in"=w307, "device index (0)"=w305, "NI-RTG Interface in"=w309) -> ("error out"=w306:errorcluster, "NI-RTG Interface out"=w308:refnum<class "NI-RTG Interface.lvclass">)  [unwired: 7 in]
              }
            }
          }
          event "send target config": Value Change {
            # "21"
            n84 = event-data() -> ()  [unwired: 1 in, 1 out]
            n85 = call-dynamic "Send Target Configuration.vi"("error in"=w319, "target config"="Target Configuration", "device index (0)"=w322, "rtg api interface"=w324) -> ("error out"=w318:errorcluster, "rtg api interface out"=w323:refnum<class "NI-RTG Interface.lvclass">)  [unwired: 5 in, 1 out]
          }
          event "send target motion": Value Change {
            # "----------------------------22----------------------------"
            n86 = event-data() -> ()  [unwired: 1 in, 1 out]
            n87 = case shown="True" w326 {
              tunnel: w336 -> [w346 w351]
              tunnel: w335 -> [w345 w348]
              tunnel: w333 -> [_ w350]
              tunnel: [w346 w349] -> w332
              tunnel: [w345 w347] -> w328
              frame False {
              }
              frame True {
                # "requires software trigger"
                n88 = call-dynamic "Send Target Configuration.vi"("error in"=w348, "target config"=T3 {"synchronization"={"synch mode"=enum."Software Trigger", "time offset (s)"=0.0}, "rtg targets"=[{"time offset (s)"=0.0, "attenuaton (dB)"=0.0, "doppler"=0.0, "target enable"=FALSE, "relative velocity enable"=FALSE}, {"time offset (s)"=0.0, "attenuaton (dB)"=0.0, "doppler"=0.0, "target enable"=FALSE, "relative velocity enable"=FALSE}, {"time offset (s)"=0.0, "attenuaton (dB)"=0.0, "doppler"=0.0, "target enable"=FALSE, "relative velocity enable"=FALSE}, {"time offset (s)"=0.0, "attenuaton (dB)"=0.0, "doppler"=0.0, "target enable"=FALSE, "relative velocity enable"=FALSE}]}, "device index (0)"=w350, "rtg api interface"=w351) -> ("error out"=w347:errorcluster, "rtg api interface out"=w349:refnum<class "NI-RTG Interface.lvclass">)  [unwired: 5 in, 1 out]
              }
            }
            n89 = call-dynamic "Send Target Configuration List - Target Motion.vi"("error in"=w328, "target motion parameters"="Target Motion Parameters", "device index (0)"=w333, "rtg api interface"=w332) -> ("error out"=w330:errorcluster, "rtg api interface out"=w331:refnum<class "NI-RTG Interface.lvclass">)  [unwired: 6 in]
            n90 = case shown="True" w325 {
              tunnel: w331 -> [w339 w344]
              tunnel: [w339 w343] -> w334
              tunnel: w330 -> [w338 w342]
              tunnel: [w338 w341] -> w327
              tunnel: w333 -> [_ w340]
              frame False {
              }
              frame True {
                n91 = call-dynamic "Send Software Trigger.vi"("error in"=w342, "device index (0)"=w340, "NI-RTG Interface in"=w344) -> ("error out"=w341:errorcluster, "NI-RTG Interface out"=w343:refnum<class "NI-RTG Interface.lvclass">)  [unwired: 7 in]
              }
            }
          }
          event "send sw trigger": Value Change {
            # "23"
            n92 = event-data() -> ()  [unwired: 1 in, 1 out]
            n93 = call-dynamic "Send Software Trigger.vi"("error in"=w354, "device index (0)"=w356, "NI-RTG Interface in"=w358) -> ("error out"=w353:errorcluster, "NI-RTG Interface out"=w357:refnum<class "NI-RTG Interface.lvclass">)  [unwired: 7 in]
          }
          event "set hardware trigger": Value Change {
            # "24"
            n94 = event-data() -> ("CtlRef"=w367:refnum<vi>)  [unwired: 1 in]
            n95 = property class="Bool (strict)"(reference=w367, "Value"=FALSE) -> ()  [unwired: 1 in, 2 out]
            n96 = local read "RTG State"() -> (w361:T1)
            n97 = case shown="Default" w361 {
              tunnel: [w370 w376] -> w365
              tunnel: w364 -> [w370 w375]
              tunnel: w363 -> [w369 w372]
              tunnel: w362 -> [_ w374]
              tunnel: [w369 w371] -> w359
              frame "Active" {
                n98 = One Button Dialog(message="Cannot set the trigger while Active.\nStop the RTG and then set the new trigger.") -> ()  [unwired: 1 in, 1 out]
              }
              frame Default {
                n99 = call-dynamic "Set Hardware Trigger.vi"("error in"=w372, "hardware trigger"="Hardware Trigger", "device index (0)"=w374, "rtg api interface"=w375) -> ("error out"=w371:errorcluster, "rtg api interface out"=w376:refnum<class "NI-RTG Interface.lvclass">)  [unwired: 6 in]
              }
            }
          }
          event "start rtg": Value Change {
            # "25"
            n100 = event-data() -> ()  [unwired: 1 in, 1 out]
            n101 = call-dynamic "Start.vi"("error in"=w378, "rtg api interface"=w381) -> ("error out"=w377:errorcluster, "rtg api interface out"=w380:refnum<class "NI-RTG Interface.lvclass">)  [unwired: 8 in]
          }
          event "stop rtg": Value Change {
            # "26"
            # "The Stop is also used to end any current file transfer or target motion operation in progress."
            n102 = event-data() -> ()  [unwired: 1 in, 3 out]
            n103 = call-dynamic "Stop.vi"("error in"=w383, "rtg api interface"=w386) -> ("error out"=w382:errorcluster, "rtg api interface out"=w385:refnum<class "NI-RTG Interface.lvclass">)  [unwired: 8 in]
          }
        }
        n104 = call-dynamic "Get RTG Status.vi"("error in"=w209, "rtg api interface"=w218) -> ("error out"=w216:errorcluster, "rtg status"=w211:string, "state"=w215:T1, "rtg api interface out"=w217:refnum<class "NI-RTG Interface.lvclass">)  [unwired: 6 in]
        n105 = Compound Arithmetic op=OR(w209, w220) -> (w210:bool)
        n106 = local write "RTG State"(w215) -> ()
        n107 = local write "RTG Status"(w211) -> ()
      }
    }
    frame #9 {
      # "31"
      # "30"
      # "28. Stop RTG\n29. Close Coprocessor Resources\n30. Close RTG\n31. Destroy RTG"
      # "28"
      # "Stop RTG, Close Hardware Resouces, and Destroy NI-RTG Object"
      n108 = call-dynamic "Stop.vi"("error in"=w389, "rtg api interface"=w395) -> ("error out"=w388:errorcluster, "rtg api interface out"=w394:refnum<class "NI-RTG Interface.lvclass">)  [unwired: 8 in]
      n109 = for {
        tunnel: w390 -> [w398] mode=indexing
        shift-right: [w396] -> w387
        shift-left: w388 -> [w397]
        # "29"
        n110 = call-dynamic "Close.vi"("error in"=w397, "rtg coprocessor link interface"=w398) -> ("error out"=w396:errorcluster)  [unwired: 9 in]
      }
      n111 = call-dynamic "Close.vi"("error in"=w387, "rtg api interface"=w394) -> ("error out"=w393:errorcluster, "rtg api interface out"=w391:refnum<class "NI-RTG Interface.lvclass">)  [unwired: 8 in]
      n112 = call-dynamic "Destroy.vi"("error in"=w393, "NI-RTG Interface in"=w391) -> ("error out"=→"Error Out":errorcluster)  [unwired: 9 in]
    }
  }
